vi "read_csv.vi"(7 "Read":bool, 11 "Read File:":path) -> (3 "File Data":T1)   [LabVIEW 2019]
uses:
  <vilib>/Analysis/Matrix/Datatypes/RealMatrix.ctl
  lib/libFileFunctions.so
  <vilib>/Analysis/Matrix/NI_Matrix.lvlib
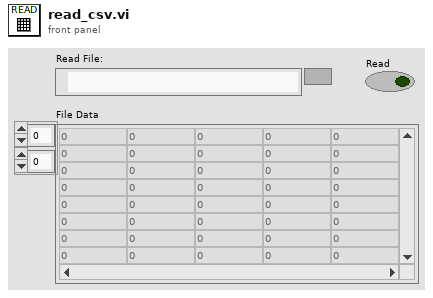
[diagram p1: front panel]
types:
  T1 = typedef "NI_Matrix.lvlib/RealMatrix.ctl" = dbl[][]
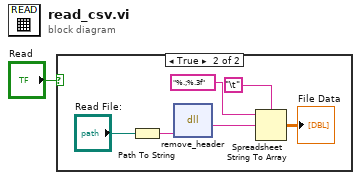
[diagram p0: block diagram]
diagram:
  n1 = case shown="True" "Read" {
    frame False {
    }
    frame True {
      n2 = Path To String(path="Read File:") -> (string=w3:string)
      n3 = dll-call lib="home/paul/Schreibtisch/Biogas_plant_setup/lib/libFileFunctions.so" fn="remove_header"("file"=w3) -> ("return type"=w2:string)  [unwired: 4 in, 2 out]
      n4 = Spreadsheet String To Array(delimiter (Tab)="\t", format string="%.;%.3f", spreadsheet string=w2) -> (array=→"File Data":dbl[][])  [unwired: 1 in]
    }
  }
